vi "sub_Format Rx Data.vi"(3 "Output Packet Array":i32[][](array[numeric])) -> (0 "Received Message":string, 1 "Array Input":u32[](array[numeric]), 2 "unsigned byte array":u8[](array[numeric]))   [LabVIEW 2023]
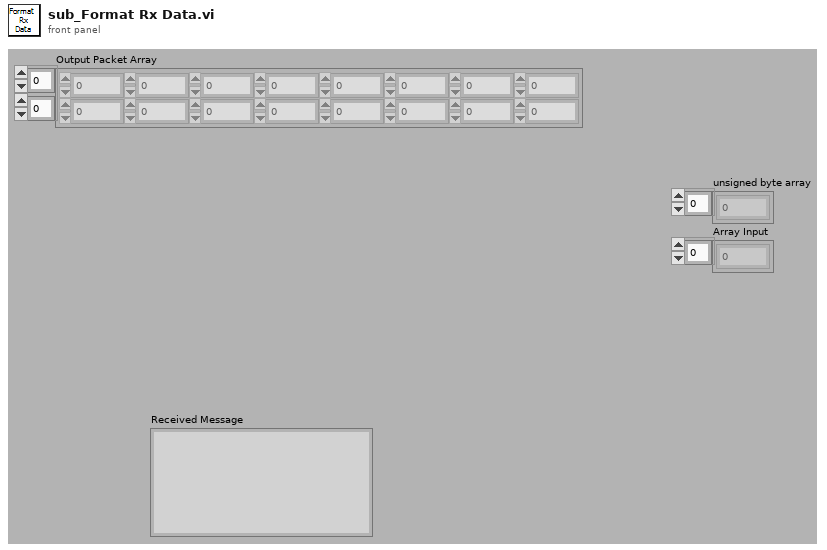
[diagram p1: front panel]
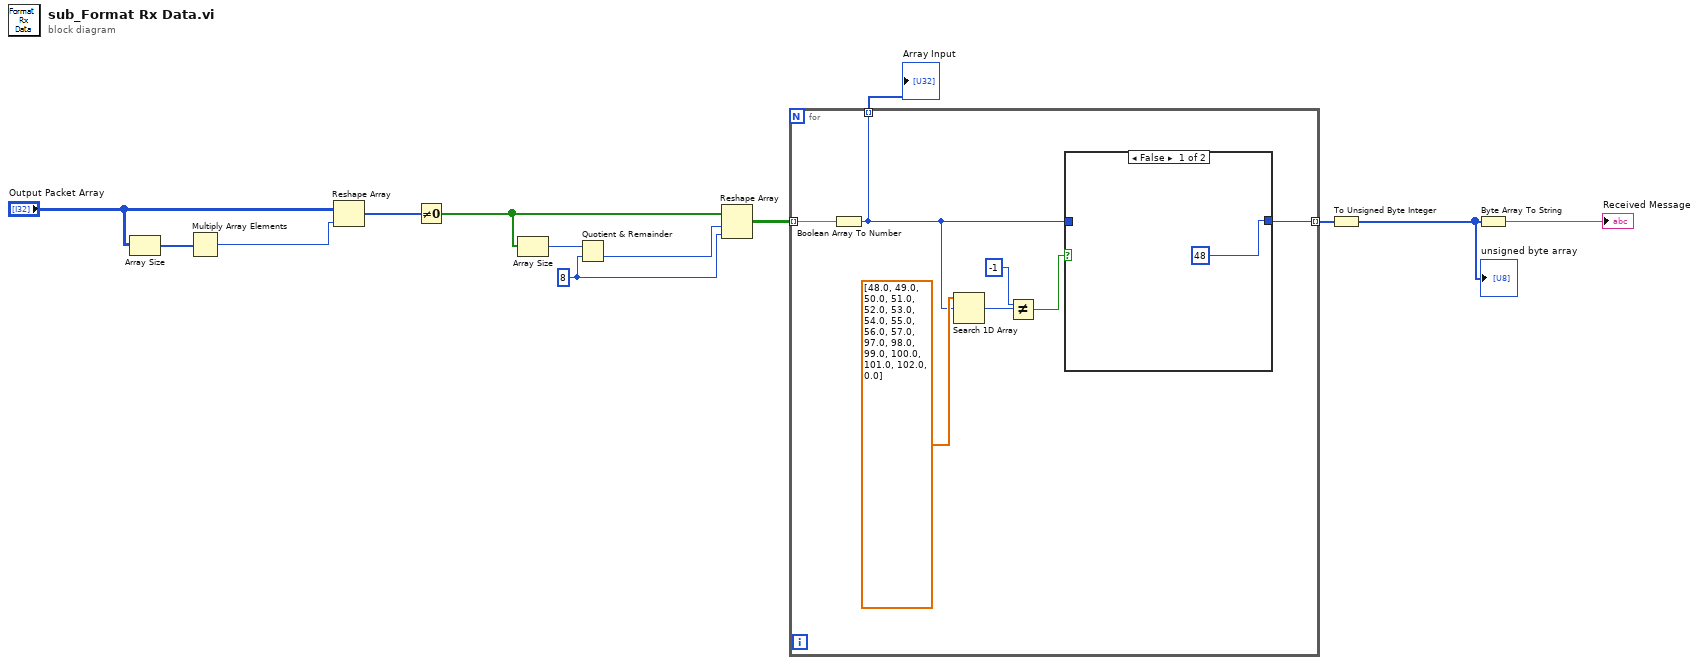
[diagram p0: block diagram]
diagram:
  w12 = 8 ("dimension size")
  n1 = Array Size(array="Output Packet Array") -> (size(s)=w6:i32[])
  n2 = Multiply Array Elements(1:w6) -> (0:w8:i32)
  n3 = Reshape Array "Reshape Array"("Output Packet Array", w8) -> (w9:i32[])
  n4 = Not Equal To 0?(x=w9) -> (x != 0?=w10:bool[])
  n5 = Array Size(array=w10) -> (size(s)=w11:i32)
  n6 = Quotient & Remainder(x=w11, y=w12) -> (floor(x/y)=w5:i32)  [unwired: 1 out]
  n7 = Reshape Array "Reshape Array"(w10, w5, w12) -> (w3:bool[][])
  n8 = for {
    tunnel: w3 -> [w20] mode=indexing
    tunnel: [w15] -> w2 mode=indexing
    tunnel: [w14] -> w1 mode=indexing
    n9 = Boolean Array To Number(Boolean array=w20) -> (number=w15:u32)
    n10 = Search 1D Array(1D array=dbl[] [48.0, 49.0, 50.0, 51.0, 52.0, 53.0, 54.0, 55.0, 56.0, 57.0, 97.0, 98.0, 99.0, 100.0, 101.0, 102.0, 0.0], element=w15) -> (index of element=w18:i32)  [unwired: 1 in]
    n11 = Not Equal?(x=-1, y=w18) -> (x != y?=w16:bool)
    n12 = case shown="False" w16 {
      tunnel: w15 -> [_ w22]
      tunnel: [48 ("x") w22] -> w14
      frame False {
      }
      frame True {
      }
    }
  }
  "Array Input" <- w2
  n13 = To Unsigned Byte Integer(number=w1) -> (unsigned 8bit integer=w4:u8[])
  "unsigned byte array" <- w4
  n14 = Byte Array To String(unsigned byte array=w4) -> (string=→"Received Message":string)
